vi "session_timeout.vi"() -> ()   [LabVIEW 2013]
doc: "Illustrates the use of timeout values for blocking functions and read operations."
uses:
  libssh2/libssh2_init_default.vi
  libssh2/libssh2.lvlib
panel:
  in  "timeout in ms (0 = indefinite)":i32
  out "error out":errorcluster
  in  "read timeout in seconds (0 = default)":i32
  out "timeout in ms":i32
  out "read timeout in seconds":i32
  # "This is the blocking timeout.\nIt defines for how long a blocking function call may wait until an error is reported.\nBy default, the timeout is zero, which means that blocking functions have no timeout (indefinite)."
  # "This is the read timeout.\nIt defines for how long a function waits for packets to arrive from the remote server.\nBy default, the timeout is 60 seconds."
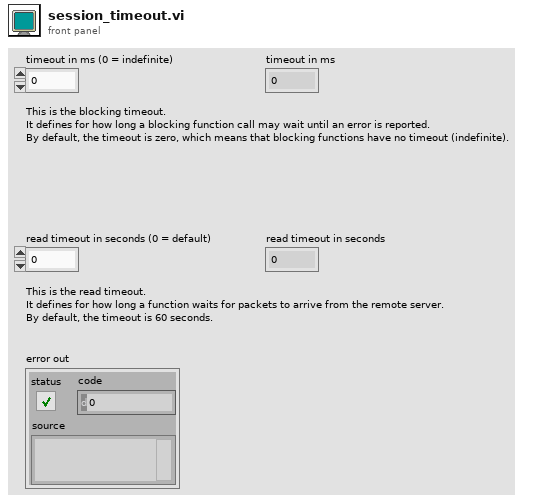
[diagram p1: front panel]
types:
  T1 = typedef "libssh2.lvlib/Session Refnum.ctl" = refnum<k1>
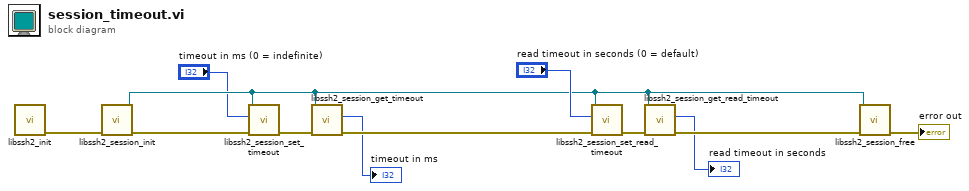
[diagram p0: block diagram]
diagram:
  n1 = call-poly "libssh2_init.vi"() -> ("error out"=w12:errorcluster)  [unwired: 11 in]
  n2 = call "libssh2_session_init.vi"("error in (no error)"=w12) -> ("error out"=w9:errorcluster, "session"=w2:T1)  [unwired: 9 in]
  n3 = call "libssh2_session_set_timeout.vi"("error in (no error)"=w9, "timeout in ms (0 = indefinite)"="timeout in ms (0 = indefinite)", "session"=w2) -> ("error out"=w3:errorcluster)  [unwired: 8 in]
  n4 = call "libssh2_session_get_timeout.vi"("error in (no error)"=w3, "session"=w2) -> ("error out"=w8:errorcluster, "timeout in ms"=→"timeout in ms":i32)  [unwired: 8 in]
  n5 = call "libssh2_session_set_read_timeout.vi"("error in (no error)"=w8, "read timeout in seconds (0 = default)"="read timeout in seconds (0 = default)", "session"=w2) -> ("error out"=w6:errorcluster)  [unwired: 8 in]
  n6 = call "libssh2_session_get_read_timeout.vi"("error in (no error)"=w6, "session"=w2) -> ("error out"=w11:errorcluster, "read timeout in seconds"=→"read timeout in seconds":i32)  [unwired: 8 in]
  n7 = call "libssh2_session_free.vi"("error in (no error)"=w11, "session"=w2) -> ("error out"=→"error out":errorcluster)  [unwired: 9 in]
